vi "Advance Settings UI.vi"(0 "Advance Setting":T2={"Prepare"={"Load SMU Output Function"=enum."VoltageSource"}, "Stimulus and Measure"={"Loop Delay"=0, "Autoset Sampling Rate?"=TRUE, "Search Tolerance (+/- % of Freq.)"=0.0}}, 11 "error in (no error)":errorcluster) -> (4 "Advance Setting Out":T2={"Prepare"={"Load SMU Output Function"=enum."VoltageSource"}, "Stimulus and Measure"={"Loop Delay"=0, "Autoset Sampling Rate?"=TRUE, "Search Tolerance (+/- % of Freq.)"=0.0}}, 15 "error out":errorcluster)   [LabVIEW 2020, in "LDO PSRR.lvlib"]
uses:
  LDO PSRR.lvlib
  Typedefs/Advance Test Input.ctl
  Reusables/Instrument APIs/Load Output Function.ctl
  <vilib>/Utility/error.llb/DialogType.ctl
  <userlib>/_Soliton/Measurement Suite/Reusables/Queue Driver/Plugin Queue Driver.lvlib
  <userlib>/_Soliton/Measurement Suite/Reusables/Plugin Common/Plugin Common.lvlib
panel:
  in  "Autoset Sampling Rate?":bool=TRUE
  in  "Output Function":T1
  in  "CLOSE":bool
  in  "Search Tolerance (+/- % of Freq.)":dbl=5.0
  in  "Loop Delay (ms)":u32 caption="Delay between Stimulus and Measure (ms)" format="%#_6p"
  in  "Panel Close":bool
  out "Banner":picture caption="Advance Settings"
  # "Load SMU"
  # "For Each Frequency"
  # "Oscilloscope"
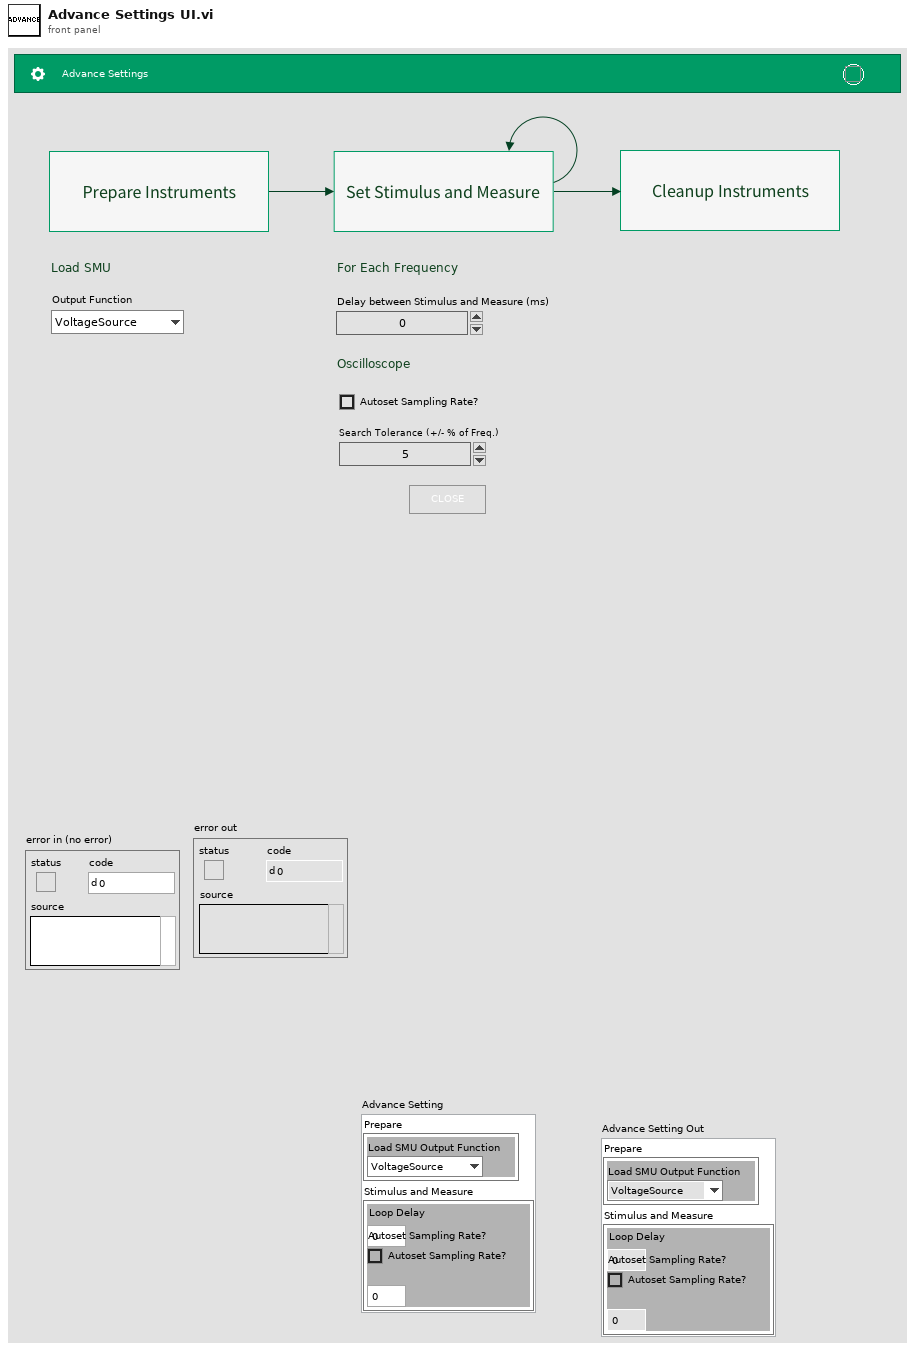
[diagram p1: front panel]
types:
  T1 = typedef "Load Output Function.ctl" = enum16{"VoltageSource", "CurrentSource"}
  T2 = typedef "LDO PSRR.lvlib/Advance Test Input.ctl" = cluster{"Prepare":cluster{"Load SMU Output Function":T1}, "Stimulus and Measure":cluster{"Loop Delay":u32, "Autoset Sampling Rate?":bool, "Search Tolerance (+/- % of Freq.)":dbl}}
  T3 = typedef "DialogType.ctl" = u16
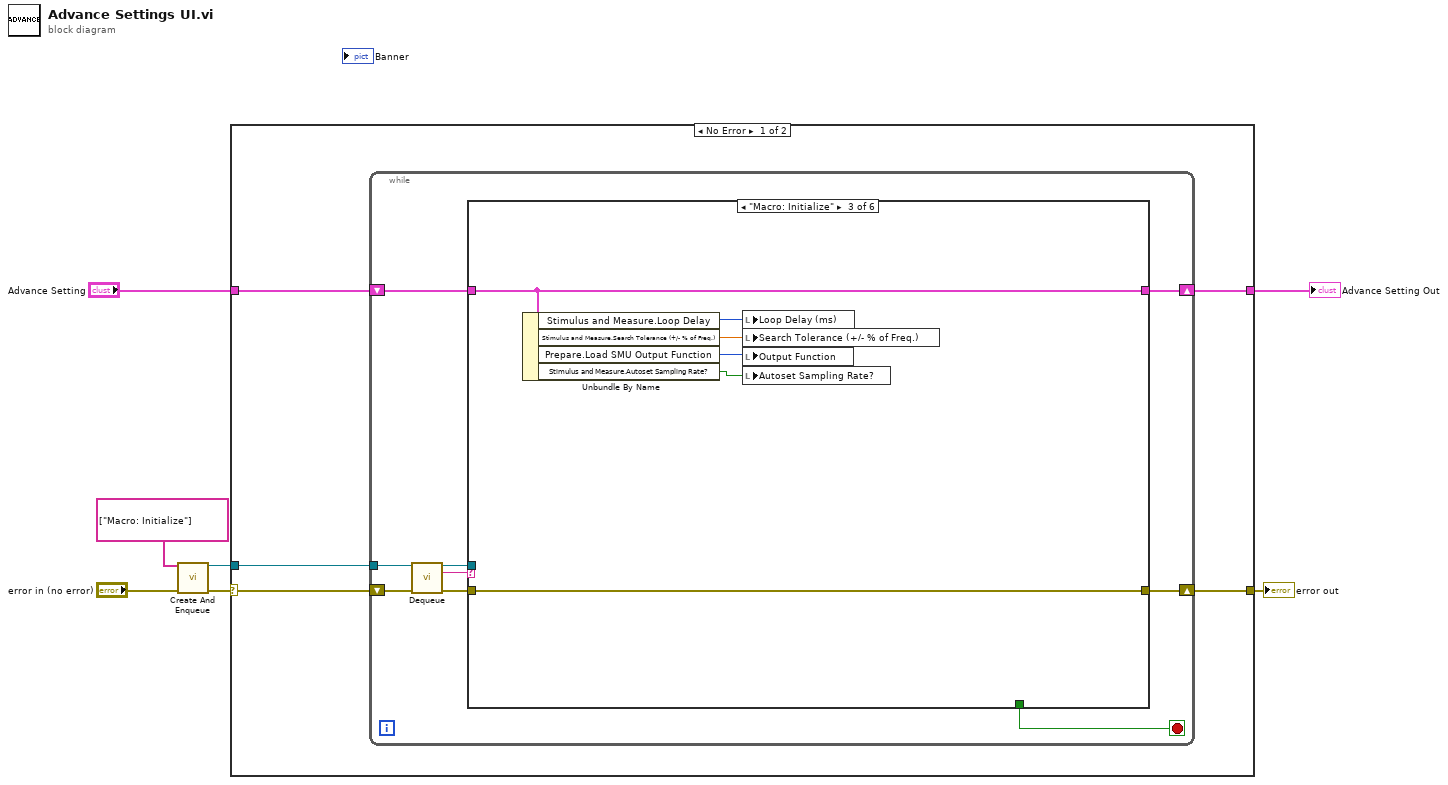
[diagram p0: block diagram]
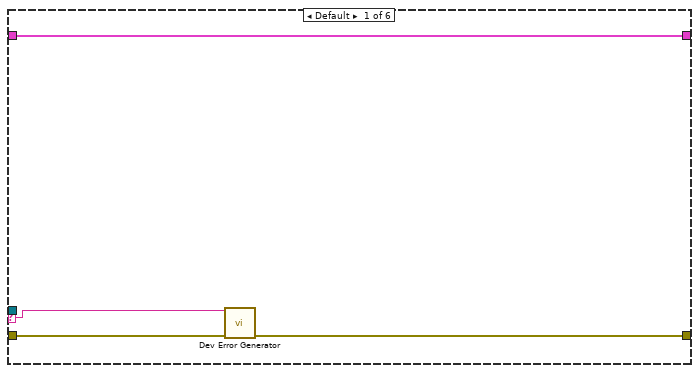
[diagram p2: hidden frame]
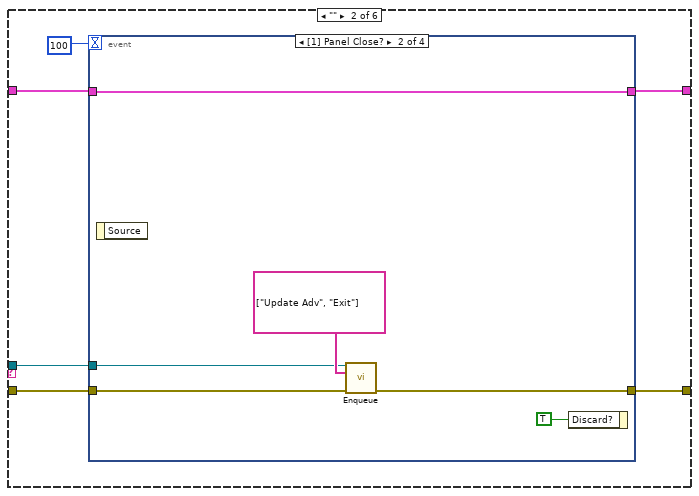
[diagram p3: hidden frame]
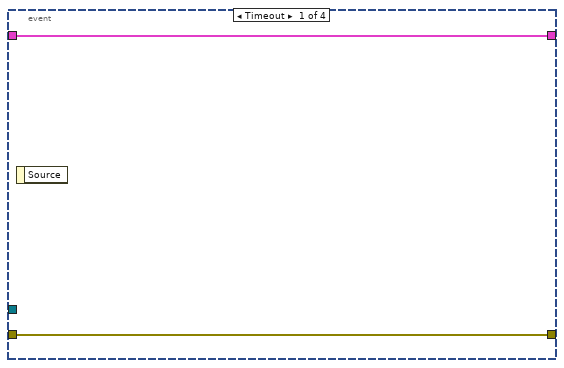
[diagram p4: hidden frame]
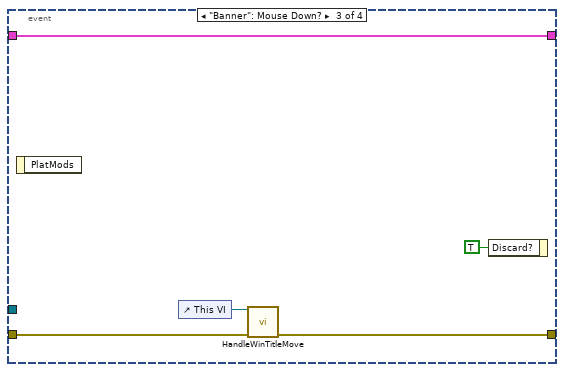
[diagram p5: hidden frame]
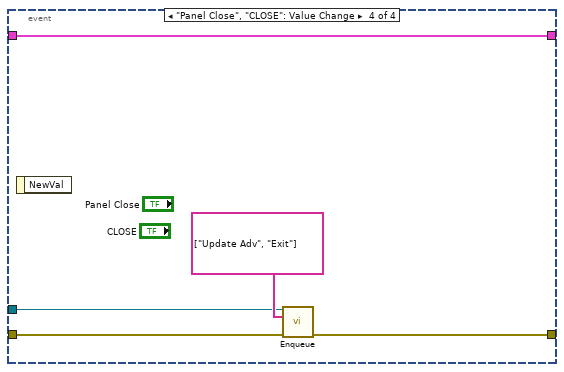
[diagram p6: hidden frame]
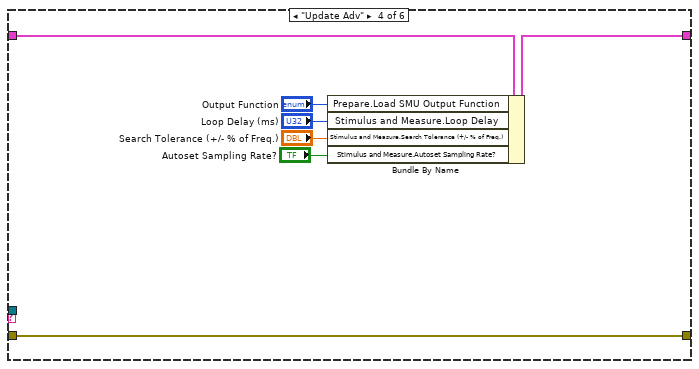
[diagram p7: hidden frame]
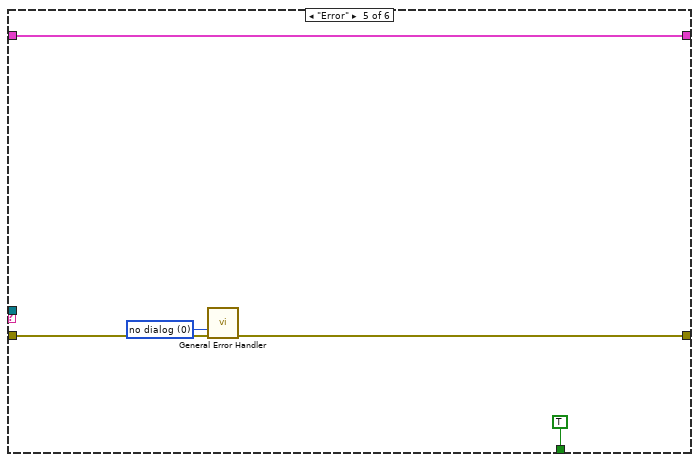
[diagram p8: hidden frame]
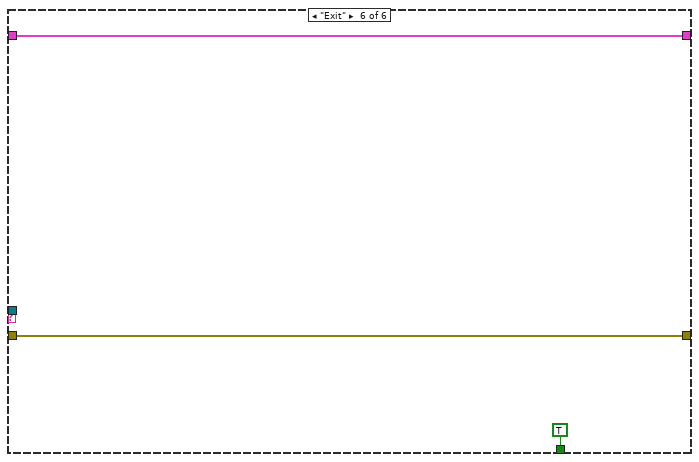
[diagram p9: hidden frame]
diagram:
  n1 = call <userlib>:"Create And Enqueue.vi"("Initial States"=string[] ["Macro: Initialize"], "error in (no error)"="error in (no error)") -> ("Queue out"=w4:refnum<queue>, "error out"=w5:errorcluster)  [unwired: 12 in]
  n2 = case shown="No Error" w5 {
    selector: w5 -> [w8 w72]
    tunnel: [w12 w72] -> w7
    tunnel: "Advance Setting" -> [w11 w71]
    tunnel: [w10 w71] -> w1
    tunnel: w4 -> [w9 _]
    frame No Error {
      n3 = while {
        tunnel: w9 -> [w18]
        shift-right: [w19] -> w10
        shift-left: w11 -> [w20]
        shift-right: [w21] -> w12
        shift-left: w8 -> [w17]
        stop <- w14 stop-if-true
        n4 = call <userlib>:"Dequeue.vi"("Queue in"=w18, "error in (no error)"=w17) -> ("Queue out"=w13:refnum<queue>, "Dequeued State"=w15:string, "error out"=w16:errorcluster)  [unwired: 11 in]
        n5 = case shown="\"Macro: Initialize\"" w15 {
          selector: w15 -> [w22 _ _ _ _ _]
          tunnel: [w24 w31 w55 w62 w65 w70] -> w21
          tunnel: w20 -> [w25 w30 w54 w60 w67 w68]
          tunnel: [w25 w29 w54 w61 w67 w68] -> w19
          tunnel: w16 -> [w23 w28 w55 w62 w64 w70]
          tunnel: [_ _ _ _ TRUE TRUE ("Discard?")] -> w14
          tunnel: w13 -> [_ w26 _ _ _ _]
          frame Default {
            n6 = call <userlib>:"Dev Error Generator.vi"("State"=w22, "error in (no error)"=w23) -> ("error out"=w24:errorcluster)  [unwired: 13 in]
          }
          frame "" {
            n7 = event shown="[1] Panel Close?" {
              selector: _ -> [_ _ _ _]
              dyn-events: _ -> [_ _ _ _]
              timeout: 100 -> [_ _ _ _]
              tunnel: w28 -> [w33 w35 w41 w46]
              tunnel: [w33 w36 w42 w47] -> w31
              tunnel: w30 -> [w32 w39 w44 w49]
              tunnel: [w32 w39 w44 w49] -> w29
              tunnel: w26 -> [_ w34 _ w45]
              event Timeout {
                n8 = event-data() -> ()  [unwired: 1 in, 1 out]
              }
              event Panel Close? {
                n9 = event-data() -> ()  [unwired: 1 in, 1 out]
                n10 = call <userlib>:"Enqueue.vi"("Queue in"=w34, "States"=string[] ["Update Adv", "Exit"] ("Initial States"), "error in (no error)"=w35) -> ("error out"=w36:errorcluster)  [unwired: 11 in, 1 out]
                n11 = event-data("Discard?"=TRUE) -> ()  [unwired: 1 in, 1 out]
              }
              event "Banner": Mouse Down? {
                n12 = event-data() -> ()  [unwired: 1 in, 1 out]
                n13 = control-ref of="This VI"() -> (w40:refnum<vi>)
                n14 = call "HandleWinTitleMove.vi"("VI in"=w40, "error in (no error)"=w41) -> ("error out"=w42:errorcluster)  [unwired: 12 in, 1 out]
                n15 = event-data("Discard?"=TRUE) -> ()  [unwired: 1 in, 1 out]
              }
              event "Panel Close", "CLOSE": Value Change {
                n16 = event-data() -> ()  [unwired: 1 in, 1 out]
                n17 = call <userlib>:"Enqueue.vi"("Queue in"=w45, "States"=string[] ["Update Adv", "Exit"] ("Initial States"), "error in (no error)"=w46) -> ("error out"=w47:errorcluster)  [unwired: 11 in, 1 out]
              }
            }
          }
          frame "Macro: Initialize" {
            n18 = Unbundle By Name(w54) -> ("Stimulus and Measure.Loop Delay"=w53:u32, "Stimulus and Measure.Search Tolerance (+/- % of Freq.)"=w52:dbl, "Prepare.Load SMU Output Function"=w51:T1, "Stimulus and Measure.Autoset Sampling Rate?"=w50:bool)
            n19 = local write "Loop Delay (ms)"(w53) -> ()
            n20 = local write "Search Tolerance (+/- % of Freq.)"(w52) -> ()
            n21 = local write "Output Function"(w51) -> ()
            n22 = local write "Autoset Sampling Rate?"(w50) -> ()
          }
          frame "Update Adv" {
            n23 = Bundle By Name(cluster=w60, "Prepare.Load SMU Output Function"="Output Function", "Stimulus and Measure.Loop Delay"="Loop Delay (ms)", "Stimulus and Measure.Search Tolerance (+/- % of Freq.)"="Search Tolerance (+/- % of Freq.)", "Stimulus and Measure.Autoset Sampling Rate?"="Autoset Sampling Rate?") -> (w61:T2)
          }
          frame "Error" {
            w66 = T3 0 items=["no dialog", "OK message", "continue or stop message", "OK message + warnings", "continue/stop + warnings"] ("type of dialog (OK msg:1)")
            n24 = call <vilib>:"General Error Handler.vi"("type of dialog (OK msg:1)"=w66, "error in (no error)"=w64) -> ("error out"=w65:errorcluster)  [unwired: 9 in, 4 out]
          }
          frame "Exit" {
          }
        }
      }
    }
    frame Error {
    }
  }
  "error out" <- w7
  "Advance Setting Out" <- w1
